vi "Handle.vi"(8 "error in (no error)":errorcluster, 11 "Acquisition in":refnum<class "Acquisition.lvclass">) -> (0 "error out":errorcluster, 3 "Acquisition out":refnum<class "Acquisition.lvclass">)   [LabVIEW 2018, in "Acquisition.lvclass"]
uses:
  Acquisition.lvclass
  Acquisition.lvclass/Acquisition.ctl
  Interface/Interface.lvclass/Interface.ctl
  Device/Device.lvclass/Device.ctl
  Channel/Channel.lvclass
  C:/Users/observer/Desktop/Sparc4GUI/Versao ZeroMQ/SPARC4_GUI - Desenv/Device/Device.lvclass
  Server/Server.lvclass
  Comm/Stream/Stream.lvclass
  Interface/Interface.lvclass
  Device/Device.lvclass
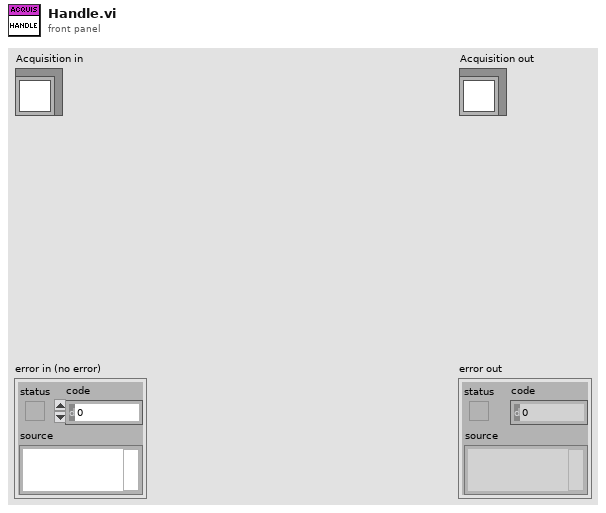
[diagram p1: front panel]
types:
  T1 = cluster{"ACQUISITION_MODE":u8, "TRIGGER_MODE":u8, "READ_MODE":u8, "PREAMP":u8, "READOUT_RATE":u8, "VERTICAL_SHIFT_SPEED":u8, "EM_MODE":u8, "EM_GAIN":u16, "SHUTTER_MODE":u8, "SHUTTER_TTL":u8, "SHUTTER_OPENING_TIME":u16, "SHUTTER_CLOSING_TIME":u16, "VBIN":u16, "HBIN":u16, "INITIAL_LINE":u16, "INITIAL_COLUMN":u16, "FINAL_LINE":u16, "FINAL_COLUMN":u16, "FRAME_TRANSFER":bool, "VERTICAL_CLOCK_VOLTAGE":u8, "AD_CHANNEL":u32}
  T2 = cluster{"ACQUISITION_MODE":bool, "TRIGGER_MODE":bool, "READ_MODE":bool, "PREAMP":bool, "READOUT_RATE":bool, "VERTICAL_SHIFT_SPEED":bool, "EM_MODE":bool, "EM_GAIN":bool, "SHUTTER_MODE":bool, "SHUTTER_TTL":bool, "SHUTTER_OPENING_TIME":bool, "SHUTTER_CLOSING_TIME":bool, "VBIN":bool, "HBIN":bool, "INITIAL_LINE":bool, "INITIAL_COLUMN":bool, "FINAL_LINE":bool, "FINAL_COLUMN":bool, "FRAME_TRANSFER":bool, "VERTICAL_CLOCK_VOLTAGE":bool, "AD_CHANNEL":bool}
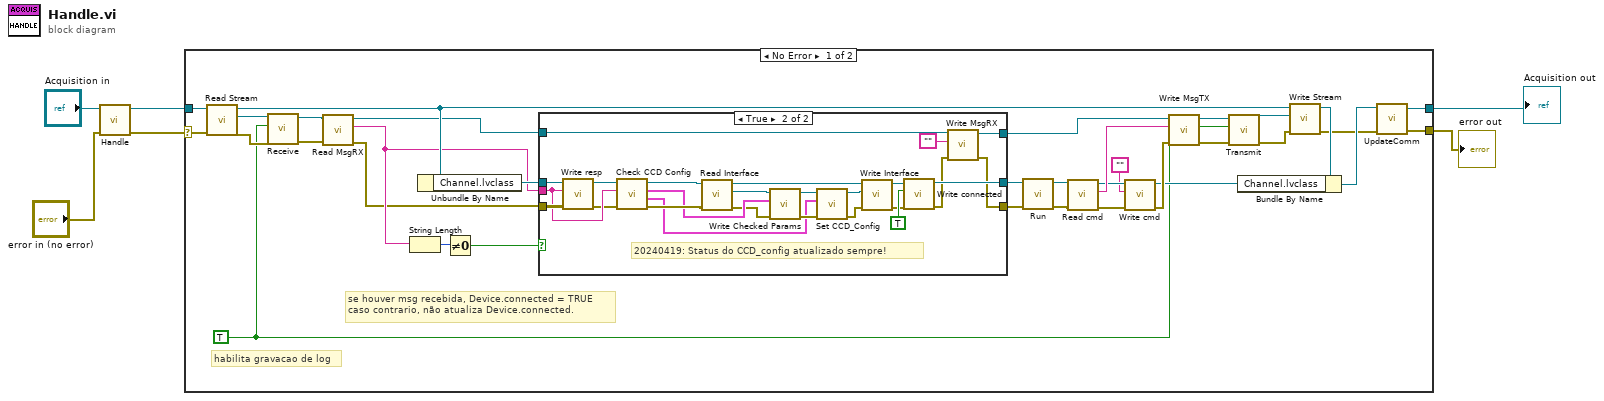
[diagram p0: block diagram]
diagram:
  n1 = call-parent "Handle.vi"("error in (no error)"="error in (no error)", "Server in"="Acquisition in") -> ("error out"=w3:errorcluster, "Server out"=w4:refnum<class "Acquisition.lvclass">)  [unwired: 8 in]
  n2 = case shown="No Error" w3 {
    selector: w3 -> [w37 w70]
    tunnel: [w12 w70] -> w1
    tunnel: [w14 w69] -> w2
    tunnel: w4 -> [w40 w69]
    frame No Error {
      w11 = TRUE ("log?")
      # "habilita gravacao de log"
      # "se houver msg recebida, Device.connected = TRUE\ncaso contrario, não atualiza Device.connected."
      n3 = call-dynamic "Read Stream.vi"("error in (no error)"=w37, "Server in"=w40) -> ("error out"=w38:errorcluster, "Stream.lvclass"=w39:refnum<class "Stream.lvclass">, "Server out"=w31:refnum<class "Acquisition.lvclass">)  [unwired: 7 in]
      n4 = call-dynamic "Receive.vi"("error in (no error)"=w38, "log?"=w11, "Stream in"=w39) -> ("error out"=w36:errorcluster, "Stream out"=w35:refnum<class "Stream.lvclass">)  [unwired: 7 in]
      n5 = call-dynamic "Read MsgRX.vi"("error in (no error)"=w36, "Comm in"=w35) -> ("error out"=w18:errorcluster, "MsgRX"=w19:string, "Comm out"=w10:refnum<class "Stream.lvclass">)  [unwired: 7 in]
      n6 = String Length(string=w19) -> (length=w25:i32)
      n7 = Unbundle By Name(w31) -> ("Channel.lvclass"=w20:refnum<class "Channel.lvclass">)
      n8 = Not Equal To 0?(x=w25) -> (x != 0?=w17:bool)
      n9 = case shown="True" w17 {
        tunnel: w18 -> [w42 w56]
        tunnel: w20 -> [w43 w66]
        tunnel: [w43 w68] -> w24
        tunnel: [w42 w54] -> w23
        tunnel: w19 -> [_ w50]
        tunnel: w10 -> [w41 w65]
        tunnel: [w41 w64] -> w9
        frame False {
        }
        frame True {
          # "20240419: Status do CCD_config atualizado sempre!"
          n10 = call-dynamic "Write resp.vi"("error in (no error)"=w56, "resp"=w50, "Device in"=w66) -> ("error out"=w49:errorcluster, "Device out"=w51:refnum<class "Channel.lvclass">)  [unwired: 7 in]
          n11 = call-dynamic "Check CCD Config.vi"("error in (no error)"=w49, "Status"=w50, "Channel in"=w51) -> ("error out"=w47:errorcluster, "cluster RX"=w44:T1, "Cluster COMPARE"=w46:T2, "Channel out"=w48:refnum<class "Channel.lvclass">)  [unwired: 5 in]
          n12 = call-dynamic "Read Interface.vi"("error in (no error)"=w47, "Channel in"=w48) -> ("error out"=w45:errorcluster, "Interface.lvclass"=w52:refnum<class "Interface.lvclass">, "Channel out"=w62:refnum<class "Channel.lvclass">)  [unwired: 7 in]
          n13 = call "Write Checked Params.vi"("error in (no error)"=w45, "Checked Params"=w46, "Interface in"=w52) -> ("error out"=w60:errorcluster, "Interface out"=w61:refnum<class "Interface.lvclass">)  [unwired: 7 in]
          n14 = call-dynamic "Set CCD_Config.vi"("error in (no error)"=w60, "input cluster"=w44, "Interface in"=w61) -> ("error out"=w59:errorcluster, "Interface out"=w53:refnum<class "Interface.lvclass">)  [unwired: 7 in]
          n15 = call-dynamic "Write Interface.vi"("error in (no error)"=w59, "Interface.lvclass"=w53, "Channel in"=w62) -> ("error out"=w58:errorcluster, "Channel out"=w57:refnum<class "Channel.lvclass">)  [unwired: 7 in]
          n16 = call "Write connected.vi"("error in (no error)"=w58, "connected"=TRUE, "Device in"=w57) -> ("error out"=w55:errorcluster, "Device out"=w68:refnum<class "Channel.lvclass">)  [unwired: 7 in]
          n17 = call-dynamic "Write MsgRX.vi"("error in (no error)"=w55, "MsgRX"="", "Comm in"=w65) -> ("error out"=w54:errorcluster, "Comm out"=w64:refnum<class "Stream.lvclass">)  [unwired: 7 in]
        }
      }
      n18 = call-dynamic "Run.vi"("error in (no error)"=w23, "Channel in"=w24) -> ("error out"=w7:errorcluster, "Channel out"=w8:refnum<class "Channel.lvclass">)  [unwired: 8 in]
      n19 = call-dynamic "Read cmd.vi"("error in (no error)"=w7, "Device in"=w8) -> ("error out"=w27:errorcluster, "cmd"=w34:string, "Device out"=w28:refnum<class "Channel.lvclass">)  [unwired: 7 in]
      n20 = call-dynamic "Write cmd.vi"("error in (no error)"=w27, "cmd"="", "Device in"=w28) -> ("error out"=w22:errorcluster, "Device out"=w21:refnum<class "Channel.lvclass">)  [unwired: 7 in]
      n21 = call-dynamic "Write MsgTX.vi"("error in (no error)"=w22, "MsgTX"=w34, "Comm in"=w9) -> ("error out"=w32:errorcluster, "Comm out"=w33:refnum<class "Stream.lvclass">)  [unwired: 7 in]
      n22 = call-dynamic "Transmit.vi"("error in (no error)"=w32, "log?"=w11, "Stream in"=w33) -> ("error out"=w29:errorcluster, "Stream out"=w30:refnum<class "Stream.lvclass">)  [unwired: 7 in]
      n23 = call-dynamic "Write Stream.vi"("error in (no error)"=w29, "Stream.lvclass"=w30, "Server in"=w31) -> ("error out"=w13:errorcluster, "Server out"=w16:refnum<class "Acquisition.lvclass">)  [unwired: 7 in]
      n24 = Bundle By Name(cluster=w16, "Channel.lvclass"=w21) -> (w15:refnum<class "Acquisition.lvclass">)
      n25 = call-dynamic "UpdateComm.vi"("error in (no error)"=w13, "Acquisition in"=w15) -> ("error out"=w12:errorcluster, "Acquisition out"=w14:refnum<class "Acquisition.lvclass">)  [unwired: 8 in]
    }
    frame Error {
    }
  }
  "error out" <- w1
  "Acquisition out" <- w2
